vi "BinarySearch1.vi"(4 "ExistingWts 1D Array":dbl[](array[numeric]), 8 "Desired Angle (degrees)":dbl, 9 "Desired Weight":dbl, 10 "Angles 1D Array":dbl[](array[numeric]), 11 "Weights 1D Array":dbl[](array[numeric])) -> (2 "Closest Angle 1":dbl, 3 "Closest Weight 1":dbl)   [LabVIEW 2012]
panel:
  out "angles-mid":i32
  out "wts-mid":i32
  out "angles-bottom":i32
  out "wts-bottom":i32
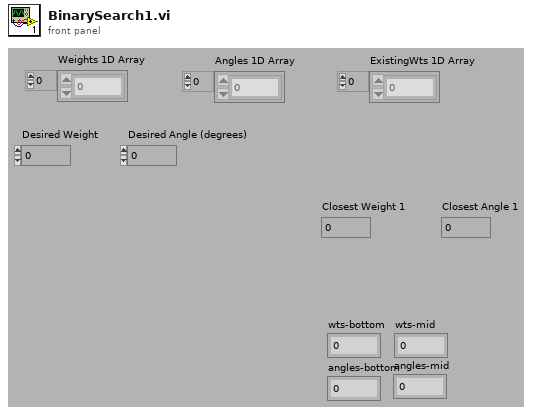
[diagram p1: front panel]
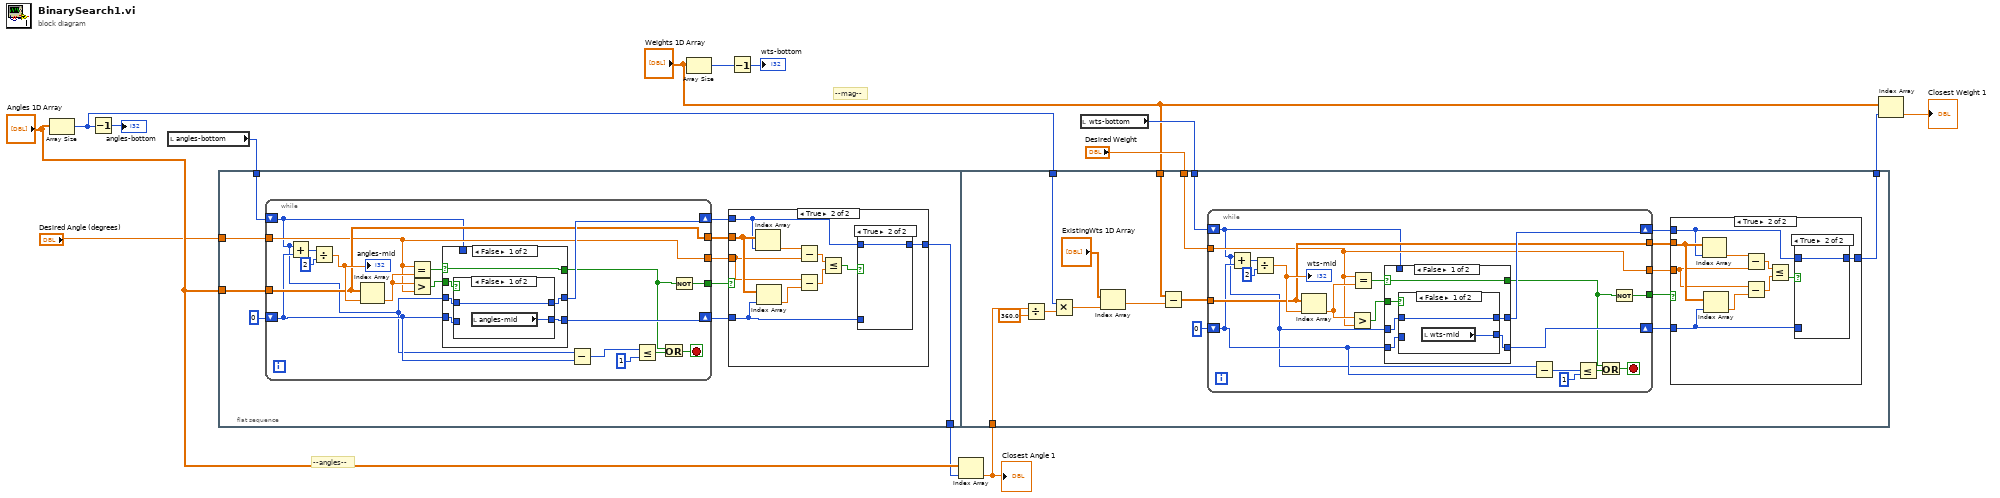
[diagram p0: block diagram]
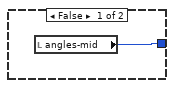
[diagram p2: hidden frame]
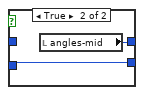
[diagram p4: hidden frame]
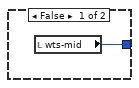
[diagram p6: hidden frame]
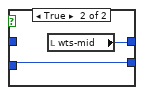
[diagram p8: hidden frame]
diagram:
  # "--angles--"
  # "--mag--"
  n1 = Array Size(array="Angles 1D Array") -> (size(s)=w2:i32)
  n2 = Decrement(x=w2) -> (x-1=→"angles-bottom":i32)
  n3 = local read "angles-bottom"() -> (w9:i32)
  n4 = flat-sequence {
    tunnel: "Angles 1D Array" -> [w24]
    tunnel: w9 -> [w23]
    tunnel: [w18] -> w8
    tunnel: "Desired Angle (degrees)" -> [w15]
    tunnel: w6 -> [w81]
    tunnel: "Desired Weight" -> [w80]
    tunnel: "Weights 1D Array" -> [w71]
    tunnel: [w78] -> w4
    tunnel: w3 -> [w74]
    tunnel: w2 -> [w76]
    frame #0 {
      n5 = while {
        tunnel: w15 -> [w44]
        tunnel: w24 -> [w45]
        shift-right: [w47] -> w21
        shift-left: 0 ("angles-bottom") -> [w43]
        shift-right: [w48] -> w17
        shift-left: w23 -> [w41]
        tunnel: [w45] -> w20
        tunnel: [w44] -> w19
        tunnel: [w39] -> w16
        stop <- w51 stop-if-true
        n6 = Add(x=w41, y=w43) -> (x+y=w53:i32)
        n7 = Divide(x=w53, y=2) -> (x/y=w46:dbl)
        "angles-mid" <- w46
        n8 = Index Array(array=w45, index=w46) -> (element=w49:dbl)
        n9 = Equal?(x=w44, y=w49) -> (x = y?=w42:bool)
        n10 = Greater?(x=w49, y=w44) -> (0:w50:bool)
        n11 = case shown="False" w42 {
          selector: w42 -> [w56 w66]
          tunnel: w50 -> [w61 _]
          tunnel: [w60 w68] -> w48
          tunnel: [w59 w67] -> w47
          tunnel: w41 -> [w58 _]
          tunnel: w43 -> [w57 w67]
          tunnel: [w56 w66] -> w38
          tunnel: w41 -> [_ w68]
          frame False {
            n12 = case shown="False" w61 {
              tunnel: [w62 w65] -> w60
              tunnel: w57 -> [_ w64]
              tunnel: w58 -> [w62 _]
              tunnel: [w63 w64] -> w59
              frame False {
                n13 = local read "angles-mid"() -> (w63:i32)
              }
              frame True {
                n14 = local read "angles-mid"() -> (w65:i32)
              }
            }
          }
          frame True {
          }
        }
        n15 = Subtract(x=w41, y=w43) -> (x-y=w54:i32)
        n16 = Less Or Equal?(x=w54, y=1) -> (x <= y?=w40:bool)
        n17 = Or(x=w38, y=w40) -> (x .or. y?=w51:bool)
        n18 = Not(x=w38) -> (.not. x?=w39:bool)
      }
      n19 = case shown="True" w16 {
        tunnel: w21 -> [_ w30]
        tunnel: w20 -> [_ w29]
        tunnel: w19 -> [_ w28]
        tunnel: [w25 w27] -> w18
        tunnel: w17 -> [_ w26]
        frame False {
          n20 = local read "angles-mid"() -> (w25:i32)
        }
        frame True {
          n21 = Index Array(array=w29, index=w26) -> (element=w32:dbl)
          n22 = Index Array(array=w29, index=w30) -> (element=w31:dbl)
          n23 = Subtract(x=w32, y=w28) -> (x-y=w33:dbl)
          n24 = Subtract(x=w28, y=w31) -> (x-y=w34:dbl)
          n25 = Less Or Equal?(x=w33, y=w34) -> (x <= y?=w35:bool)
          n26 = case shown="True" w35 {
            tunnel: w26 -> [_ w37]
            tunnel: w30 -> [w36 _]
            tunnel: [w36 w37] -> w27
            frame False {
            }
            frame True {
            }
          }
        }
      }
    }
    frame #1 {
      n27 = Divide(x=w74, y=360.0) -> (x/y=w77:dbl)
      n28 = Multiply(x=w76, y=w77) -> (x*y=w73:dbl)
      n29 = Index Array(array="ExistingWts 1D Array", index=w73) -> (element=w70:dbl)
      n30 = Subtract(x=w71, y=w70) -> (x-y=w69:dbl[])
      n31 = while {
        tunnel: w80 -> [w108]
        tunnel: w69 -> [w109]
        shift-right: [w111] -> w83
        shift-left: 0 -> [w107]
        shift-right: [w112] -> w85
        shift-left: w81 -> [w102]
        tunnel: [w109] -> w82
        tunnel: [w108] -> w84
        tunnel: [w100] -> w86
        stop <- w115 stop-if-true
        n32 = Add(x=w102, y=w107) -> (x+y=w117:i32)
        n33 = Divide(x=w117, y=2) -> (x/y=w110:dbl)
        "wts-mid" <- w110
        n34 = Index Array(array=w109, index=w110) -> (element=w113:dbl)
        n35 = Greater?(x=w113, y=w108) -> (0:w114:bool)
        n36 = Equal?(x=w108, y=w113) -> (x = y?=w103:bool)
        n37 = case shown="False" w103 {
          selector: w103 -> [w118 w128]
          tunnel: w114 -> [w119 _]
          tunnel: [w123 w130] -> w112
          tunnel: [w122 w129] -> w111
          tunnel: w102 -> [w121 _]
          tunnel: w107 -> [w120 w129]
          tunnel: w102 -> [_ w130]
          tunnel: [w118 w128] -> w101
          frame False {
            n38 = case shown="False" w119 {
              tunnel: [w124 w127] -> w123
              tunnel: w120 -> [_ w126]
              tunnel: w121 -> [w124 _]
              tunnel: [w125 w126] -> w122
              frame False {
                n39 = local read "wts-mid"() -> (w125:i32)
              }
              frame True {
                n40 = local read "wts-mid"() -> (w127:i32)
              }
            }
          }
          frame True {
          }
        }
        n41 = Subtract(x=w102, y=w107) -> (x-y=w106:i32)
        n42 = Less Or Equal?(x=w106, y=1) -> (x <= y?=w104:bool)
        n43 = Or(x=w101, y=w104) -> (x .or. y?=w115:bool)
        n44 = Not(x=w101) -> (.not. x?=w100:bool)
      }
      n45 = case shown="True" w86 {
        tunnel: [w87 w97] -> w78
        tunnel: w82 -> [_ w96]
        tunnel: w83 -> [_ w95]
        tunnel: w84 -> [_ w92]
        tunnel: w85 -> [_ w88]
        frame False {
          n46 = local read "wts-mid"() -> (w87:i32)
        }
        frame True {
          n47 = Index Array(array=w96, index=w88) -> (element=w93:dbl)
          n48 = Index Array(array=w96, index=w95) -> (element=w94:dbl)
          n49 = Subtract(x=w93, y=w92) -> (x-y=w91:dbl)
          n50 = Subtract(x=w92, y=w94) -> (x-y=w90:dbl)
          n51 = Less Or Equal?(x=w91, y=w90) -> (x <= y?=w89:bool)
          n52 = case shown="True" w89 {
            tunnel: w88 -> [_ w99]
            tunnel: w95 -> [w98 _]
            tunnel: [w98 w99] -> w97
            frame False {
            }
            frame True {
            }
          }
        }
      }
    }
  }
  n53 = Array Size(array="Weights 1D Array") -> (size(s)=w12:i32)
  n54 = Decrement(x=w12) -> (x-1=→"wts-bottom":i32)
  n55 = Index Array(array="Angles 1D Array", index=w8) -> (element=w3:dbl)
  "Closest Angle 1" <- w3
  n56 = local read "wts-bottom"() -> (w6:i32)
  n57 = Index Array(array="Weights 1D Array", index=w4) -> (element=→"Closest Weight 1":dbl)
